vi "get Maximum Velocity.vi"(11 "Motion in":refnum<class "Motion.lvclass">) -> (3 "Maximum Velocity":sgl=90.0 format="%.3g")   [LabVIEW 2021, in "Motion.lvclass"]
uses:
  Motion.lvclass
  Motion.lvclass/Motion.ctl
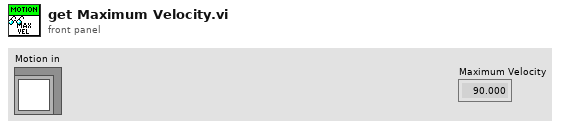
[diagram p1: front panel]
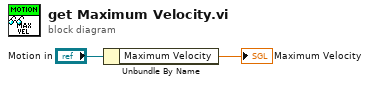
[diagram p0: block diagram]
diagram:
  n1 = Unbundle By Name("Motion in") -> ("Maximum Velocity"=→"Maximum Velocity":sgl)
